vi "j1939 main.vi"(6 "Outgoing Cyclic Cfg":T1 {"Outgoing Cyclic Frame"."Transmit Propreties"."Transmit Time" format="%#_p"}, 7 "Incoming cfg":T7, 8 "error in":errorcluster, 10 "tag bus queues":T6, 11 "J1939 internal data":T9={"J1939 XNET Settings"={"XNET Database"="", "XNET Cluster"="", "CAN port"="", "Baud rate [Bd]"=0, "J1939 Network Address"=0, "Name"=0, "Termination"=0}, "j1939 queues"={"Processed Outgoing"=refnum, "Process Outgoing"=refnum, "stop notifier"=refnum, "error queue"=refnum, "active dtc"=refnum, "processed inc"=refnum}, "fgv references"={"BAM Buffer"=refnum, "CM Buffer"=refnum, "CM Gen"=refnum, "BAM Gen"=refnum, "Address Claims"=refnum, "RQST"=refnum, "scaling lut"=refnum, "data lut"=refnum, "cyclic scheduler"=refnum}, "frame in"="", "frame out"="", "timing"={"tb to j1939 queue timeout"=100, "j1939 to tb queue timeout"=100, "dtc loop period (ms)"=100, "CAN in loop period (ms)"=100, "process incoming queue timeout (ms)"=100, "Outgoing Write Decimation"=0, "process outgoing loop rate (ms)"=0, "periodic outgoing queue timeout (ms)"=10, "CAN out queue timeout (ms)"=100}}) -> (0 "error out":errorcluster)   [LabVIEW 2013, in "J1939.lvlib"]
uses:
  J1939.lvlib
  Internals/API Types/Internal Data.ctl
  Internals/API Types/XNET Settings.ctl
  Internals/API Types/Setup Information Cluster.ctl
  Internals/API Types/CAN Outgoing Message Cluster.ctl
  Internals/API Types/Convert DTCs Cluster.ctl
  <vilib>/xnet/xnet.llb/XNET Frame CAN.ctl
  <vilib>/xnet/xnet.llb/XNET Frame Type CAN.ctl
  Internals/TP/TP List References.ctl
  Internals/BAM/BAM Buffer Connections List_Ref.ctl
  Internals/Connection Mode/Connection Mode Generation Connection Ref.ctl
  Internals/BAM/BAM Generation Connections List_Ref.ctl
  Internals/LUTs/J1939 Address Table Reference.ctl
  Internals/RQST/RQST Lookup Table Reference.ctl
  Internals/LUTs/J1939 Conversion Lookup Table Reference.ctl
  Internals/LUTs/J1939 Data Lookup Table Reference.ctl
  Internals/LUTs/Cyclic Frame Scheduler Lut Reference.ctl
  Configuration/TypeDefs/timing configuration.ctl
  Internals/CD/CD Incoming Single Point Configuration.ctl
  Internals/CD/CD Incoming Single Point Frame Pairs.ctl
  Internals/API Types/Signal Mapping.ctl
  <vilib>/NI/Tag Bus/tag/Data Type.ctl
  Internals/API Types/Tag Bus Queues.ctl
  <vilib>/NI/Tag Bus/table/data table.ctl
  Internals/CD/CD Outgoing Cyclic Configuration.ctl
  Internals/CD/CD Outgoing Cyclic Frame Pairs.ctl
  Internals/API Types/XNET Frame Event Properties.ctl
  <vilib>/NI/Tag Bus/table/data table.lvlib
  <vilib>/NI/Tag Bus/tag/tag descriptor.lvclass
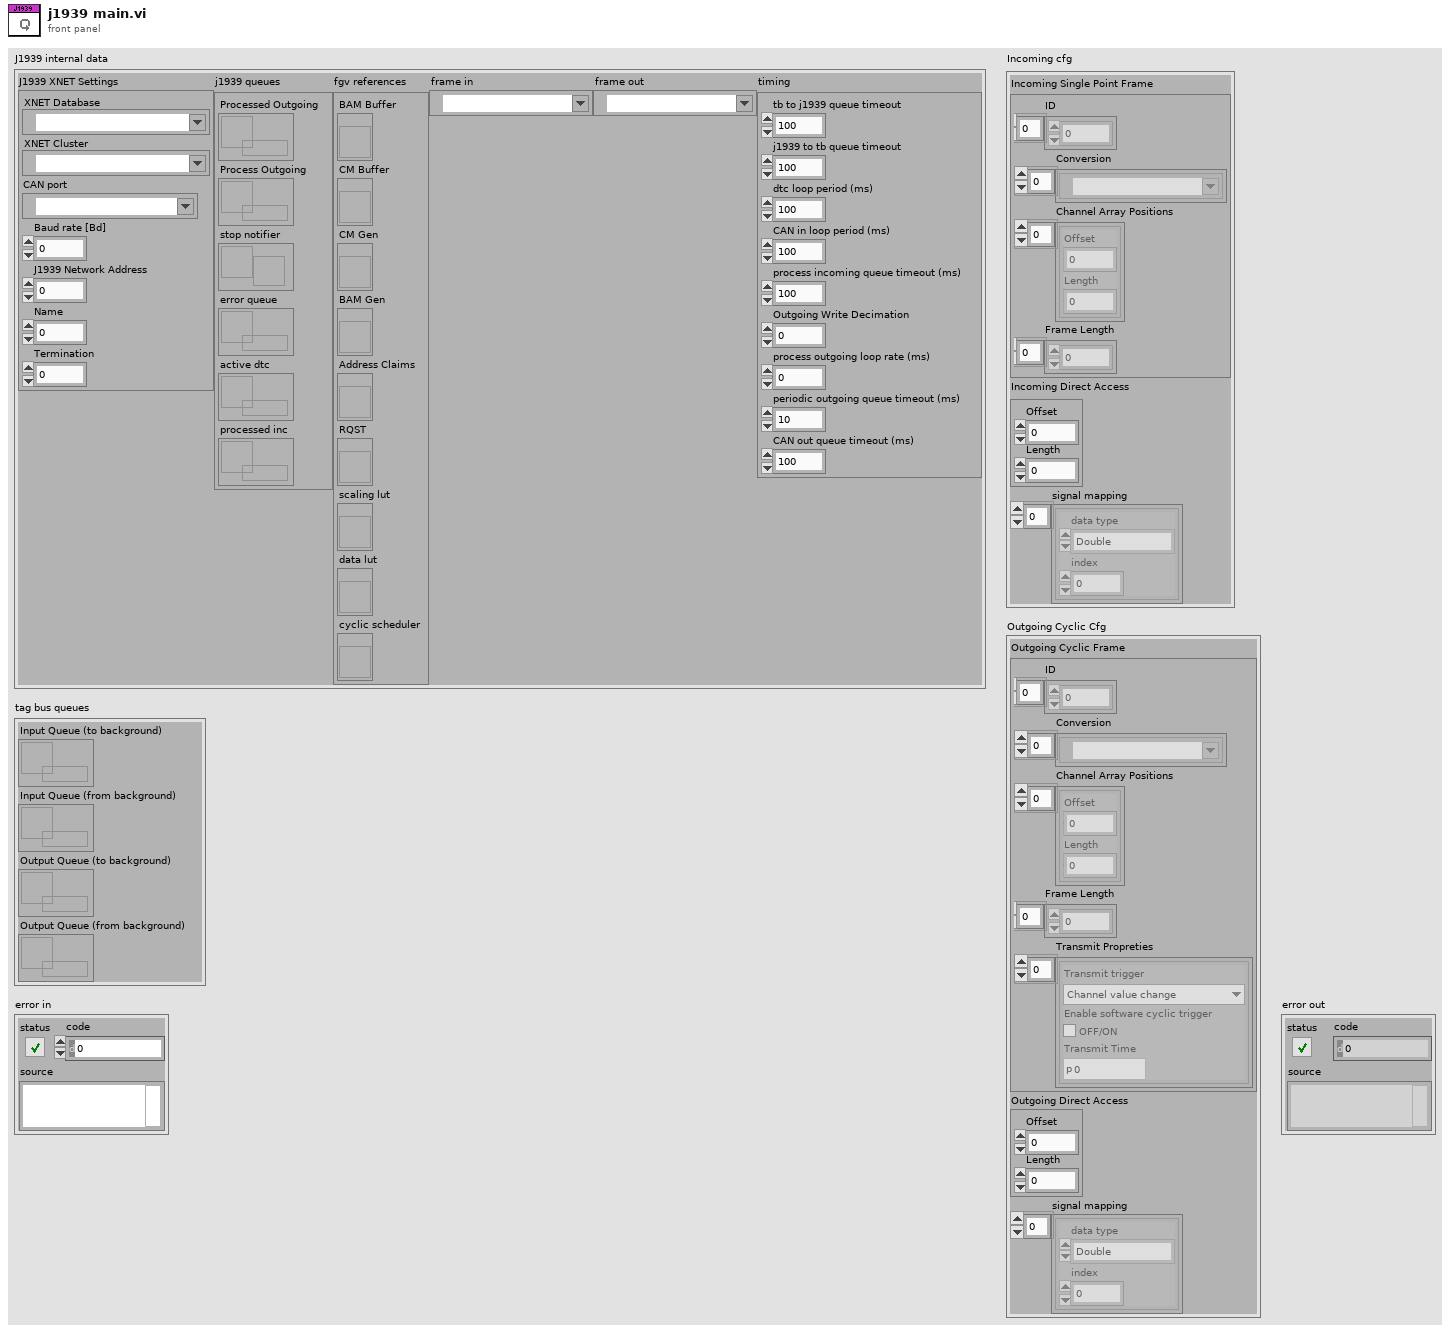
[diagram p1: front panel]
types:
  T1 = typedef "J1939.lvlib/CD Outgoing Cyclic Configuration.ctl" = cluster{"Outgoing Cyclic Frame":T2, "Outgoing Direct Access":cluster{"Offset":u32, "Length":u32}, "signal mapping":T4[]}
  T2 = typedef "J1939.lvlib/CD Outgoing Cyclic Frame Pairs.ctl" = cluster{"ID":u32[], "Conversion":refnum<k21>[], "Channel Array Positions":cluster{"Offset":u32, "Length":u32}[], "Frame Length":u32[], "Transmit Propreties":T3[]}
  T3 = typedef "J1939.lvlib/XNET Frame Event Properties.ctl" = cluster{"Transmit trigger":enum16{"Channel value change"}, "Enable software cyclic trigger":bool, "Transmit Time":dbl}
  T4 = typedef "J1939.lvlib/signal mapping.ctl" = cluster{"data type":T5, "index":i32}
  T5 = typedef "tag bus.lvlib/tag descriptor.lvclass/Data Type.ctl" = enum16{"Double", "Single", "I64", "I32", "I16", "I8", "U64", "U32", "U16", "U8", "Boolean", "String", "Array of Double", "Array of Single", "Array of I64", "Array of I32", "Array of I16", "Array of I8", "Array of U64", "Array of U32", "Array of U16", "Array of U8", "Array of Boolean", "Array of String"}
  T6 = typedef "J1939.lvlib/Tag Bus Queues.ctl" = cluster{"Input Queue (to background)":refnum<queue>, "Input Queue (from background)":refnum<queue>, "Output Queue (to background)":refnum<queue>, "Output Queue (from background)":refnum<queue>}
  T7 = typedef "J1939.lvlib/CD Incoming Single Point Configuration.ctl" = cluster{"Incoming Single Point Frame":T8, "Incoming Direct Access":cluster{"Offset":u32, "Length":u32}, "signal mapping":T4[]}
  T8 = typedef "J1939.lvlib/CD Incoming Single Point Frame Pairs.ctl" = cluster{"ID":u32[], "Conversion":refnum<k21>[], "Channel Array Positions":cluster{"Offset":u32, "Length":u32}[], "Frame Length":u32[]}
  T9 = typedef "J1939.lvlib/Internal Data.ctl" = cluster{"J1939 XNET Settings":T10, "j1939 queues":T11, "fgv references":T12, "frame in":refnum<k21>, "frame out":refnum<k21>, "timing":T21}
  T10 = typedef "J1939.lvlib/XNET settings.ctl" = cluster{"XNET Database":refnum<k21>, "XNET Cluster":refnum<k21>, "CAN port":refnum<k21>, "Baud rate [Bd]":u32, "J1939 Network Address":u8, "Name":u64, "Termination":u32}
  T11 = typedef "J1939.lvlib/Setup Information Cluster.ctl" = cluster{"Processed Outgoing":refnum<queue>, "Process Outgoing":refnum<queue>, "stop notifier":refnum<notifier>, "error queue":refnum<queue>, "active dtc":refnum<queue>, "processed inc":refnum<queue>}
  T12 = typedef "J1939.lvlib/TP List References.ctl" = cluster{"BAM Buffer":T13, "CM Buffer":T13, "CM Gen":T14, "BAM Gen":T15, "Address Claims":T16, "RQST":T17, "scaling lut":T18, "data lut":T19, "cyclic scheduler":T20}
  T13 = typedef "J1939.lvlib/BAM Buffer Connections List_Ref.ctl" = refnum<vi>
  T14 = typedef "J1939.lvlib/Connection Mode Generation Connection Ref.ctl" = refnum<vi>
  T15 = typedef "J1939.lvlib/BAM Generation Connections List_Ref.ctl" = refnum<vi>
  T16 = typedef "J1939.lvlib/J1939 Address Table Reference.ctl" = refnum<vi>
  T17 = typedef "J1939.lvlib/RQST Lookup Table Reference.ctl" = refnum<vi>
  T18 = typedef "J1939.lvlib/J1939 Conversion Lookup Table Reference.ctl" = refnum<vi>
  T19 = typedef "J1939.lvlib/J1939 Data Lookup Table Reference.ctl" = refnum<vi>
  T20 = typedef "J1939.lvlib/cyclic frame scheduler lut reference.ctl" = refnum<vi>
  T21 = typedef "J1939.lvlib/timing configuration.ctl" = cluster{"tb to j1939 queue timeout":i32, "j1939 to tb queue timeout":i32, "dtc loop period (ms)":i32, "CAN in loop period (ms)":i32, "process incoming queue timeout (ms)":i32, "Outgoing Write Decimation":u32, "process outgoing loop rate (ms)":i32, "periodic outgoing queue timeout (ms)":i32, "CAN out queue timeout (ms)":i32}
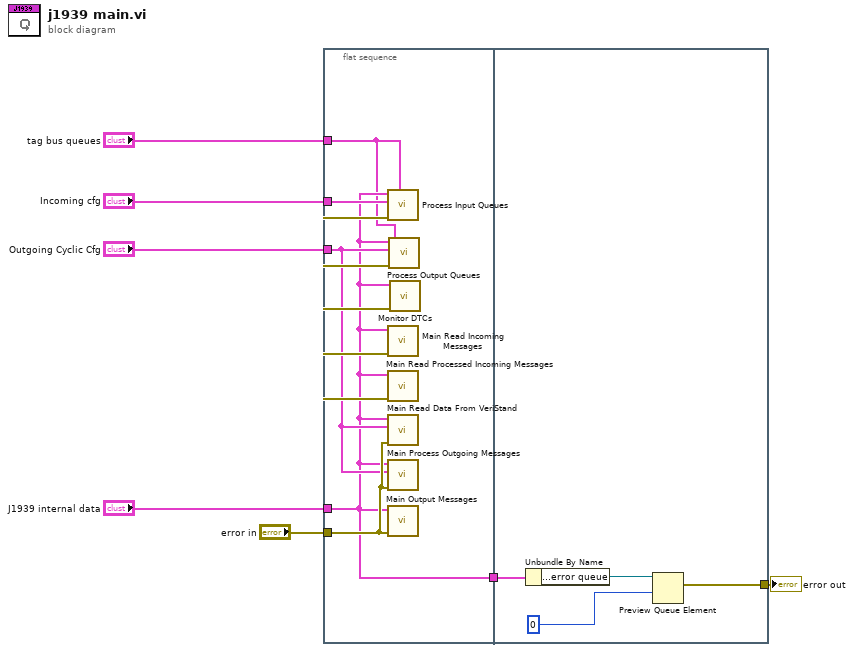
[diagram p0: block diagram]
diagram:
  n1 = flat-sequence {
    tunnel: "Incoming cfg" -> [w12]
    tunnel: "tag bus queues" -> [w8]
    tunnel: "error in" -> [w11]
    tunnel: "Outgoing Cyclic Cfg" -> [w10]
    tunnel: "J1939 internal data" -> [w9]
    tunnel: [w9] -> w1
    tunnel: [w15] -> w2
    tunnel: w1 -> [w14]
    frame #0 {
      n2 = call "Process Input Queues.vi"("tag bus queues"=w8, "error in"=w11, "Incoming cfg"=w12, "J1939 internal data"=w9) -> ()  [unwired: 8 in]
      n3 = call "Main Read Incoming Messages.vi"("error in"=w11, "internal data"=w9) -> ()  [unwired: 10 in]
      n4 = call "Main Read Processed Incoming Messages.vi"("error in"=w11, "internal data"=w9) -> ()  [unwired: 10 in]
      n5 = call "Main Read Data From VeriStand.vi"("error in"=w11, "Outgoing Cyclic Configuraiton"=w10, "internal data"=w9) -> ()  [unwired: 9 in]
      n6 = call "Main Process Outgoing Messages.vi"("error in"=w11, "Outgoing Cyclic Configuraiton"=w10, "internal data"=w9) -> ()  [unwired: 9 in]
      n7 = call "Main Output Messages.vi"("error in"=w11, "internal data"=w9) -> ()  [unwired: 10 in]
      n8 = call "Process Output Queues.vi"("tag bus queues"=w8, "error in"=w11, "Outgoing Cyclic Cfg"=w10, "J1939 internal data"=w9) -> ()  [unwired: 8 in]
      n9 = call "Monitor DTCs.vi"("error in"=w11, "J1939 internal data"=w9) -> ()  [unwired: 10 in]
    }
    frame #1 {
      n10 = Unbundle By Name(w14) -> ("j1939 queues.error queue"=w13:refnum<queue>)
      n11 = Preview Queue Element(queue=w13, timeout in ms (-1)=0) -> (element=w15:errorcluster)  [unwired: 1 in, 3 out]
    }
  }
  "error out" <- w2
